vi "S2DS_Update WC (SubVI).vi"(11 "All channel parameters (in)":T1 {"Scan parameters"."Y data taking" items=["in both direction", "in up direction only", "in down direction only"]; "Scan parameters"."X data taking" items=["in both direction", "in up direction only", "in down direction only"]}) -> (2 "Change required":i32[](array[numeric]), 3 "All channel parameters (out)":T1 {"Scan parameters"."Y data taking" items=["in both direction", "in up direction only", "in down direction only"]; "Scan parameters"."X data taking" items=["in both direction", "in up direction only", "in down direction only"]})   [LabVIEW 2025]
uses:
  TYPE DEFS/S2DS_All Channel Parameters.ctl
  TYPE DEFS/S2DS_WC info.ctl
  TYPE DEFS/S2DS_Single WC info.ctl
  TYPE DEFS/S2DS_RC info.ctl
  TYPE DEFS/S2DS_Single RC info.ctl
  TYPE DEFS/S2DS_DAC info new.ctl
  TYPE DEFS/S2DS_Single DC info.ctl
  TYPE DEFS/S2DS_Array Inst Info.ctl
  TYPE DEFS/S2DS_Sweep Info.ctl
panel:
  in  "Tab Control":enum32{"Basic", "Advanced", "Formula"}(tab)
  in  "Step 2":dbl caption="Step size"
  in  "Rate up":dbl
  in  "Rate down":dbl
  in  "Min end":dbl
  in  "Max end":dbl
  in  "Data Bin size":dbl
  in  "Target 2":dbl caption="Target"
  out "Factor":dbl
  out "Current value":dbl
  in  "Factor 2":dbl
  in  "Current value 2":dbl
  out "Factor 3":dbl caption="Factor"
  out "Current value 3":dbl caption="Present level"
  in  "Update formula":bool
  in  "Undo":bool
  in  "OK 2":bool
  in  "Select channel to edit":u16(ring) items=["A ( Unit)", "A ( Unit)", "A ( Unit)", "A ( Unit)", "A ( Unit)", "A ( Unit)", "A ( Unit)", "A ( Unit)", "A ( Unit)"]
  in  "OK":bool
  # "Update Write Channel Info..."
  # "Old value"
  # "Updated"
  # "Enter new"
  # "NOTE:  If current level is not equal to target, the\nprogram will immedietely drive the instrument."
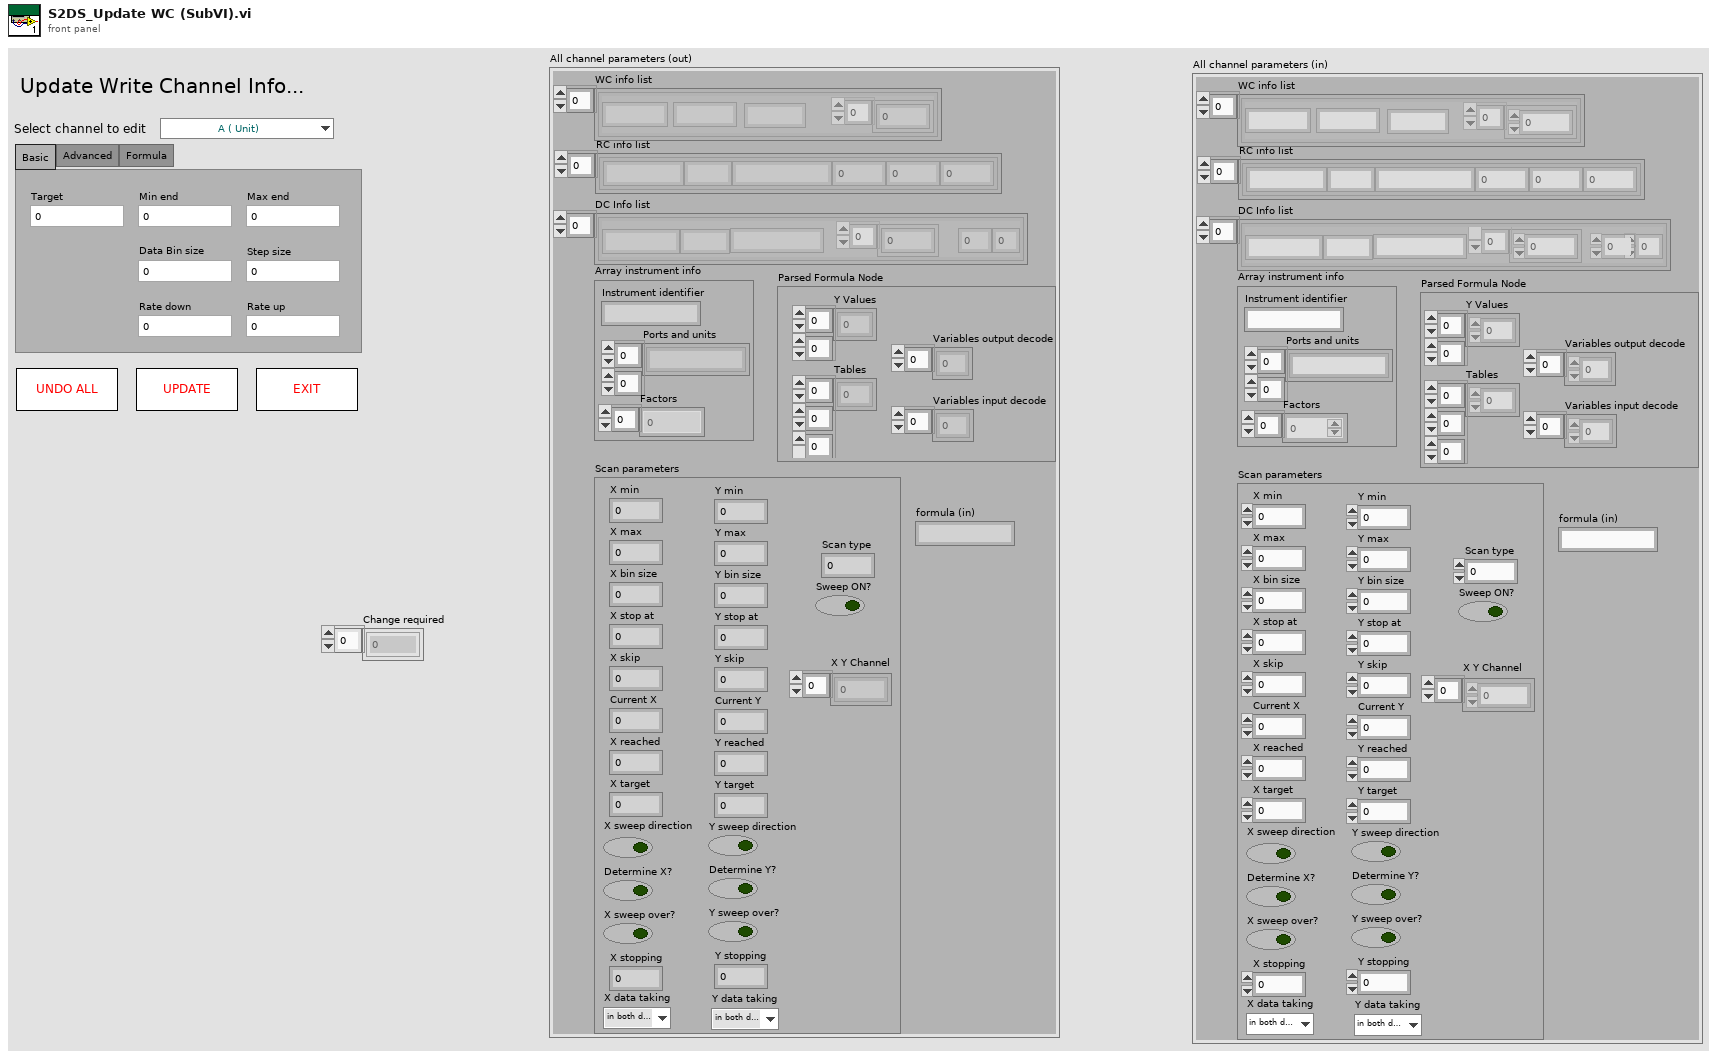
[diagram p1: front panel]
types:
  T1 = typedef "S2DS_All Channel Parameters.ctl" = cluster{"WC info list":T2, "RC info list":T4, "DC Info list":T6, "Array instrument info":T8, "Scan parameters":T9, "Parsed Formula Node":cluster{"Y Values":dbl[][], "Tables":i32[][][], "Variables input decode":i32[], "Variables output decode":i32[]}, "formula (in)":string}
  T2 = typedef "S2DS_WC info.ctl" = T3[]
  T3 = typedef "S2DS_Single WC info.ctl" = cluster{"Instrument identifier":string, "Write channel parameters":dbl[], "Name":string, "Unit":string}
  T4 = typedef "S2DS_RC info.ctl" = T5[]
  T5 = typedef "S2DS_Single RC info.ctl" = cluster{"Instrument identifier":string, "Factor":dbl, "Averaging":i32, "Wait (ms)":i32, "Unit":string, "Name":string}
  T6 = typedef "S2DS_DAC info new.ctl" = T7[]
  T7 = typedef "S2DS_Single DC info.ctl" = cluster{"Operation identifier":string, "DC parameters":dbl[], "U":i32, "V":i32, "Name":string, "Unit":string}
  T8 = typedef "S2DS_Array Inst Info.ctl" = cluster{"Instrument identifier":string, "Ports and units":string[][], "Factors":dbl[]}
  T9 = typedef "S2DS_Sweep Info.ctl" = cluster{"X min":ext, "X max":dbl, "Y min":dbl, "Y max":dbl, "X bin size":dbl, "Y bin size":dbl, "X stop at":dbl, "Y stop at":dbl, "X skip":u64, "Y skip":u64, "Current X":dbl, "Current Y":dbl, "X reached":i32, "Y reached":i32, "X target":dbl, "Y target":dbl, "Sweep ON?":bool, "X sweep direction":bool, "Y sweep direction":bool, "Determine X?":bool, "Determine Y?":bool, "X sweep over?":bool, "Y sweep over?":bool, "Scan type":i32, "X stopping":i32, "Y stopping":i32, "X Y Channel":u16[], "X data taking":u16, "Y data taking":u16}
  T10 = cluster{"Y Values":dbl[][], "Tables":i32[][][], "Variables input decode":i32[], "Variables output decode":i32[]}
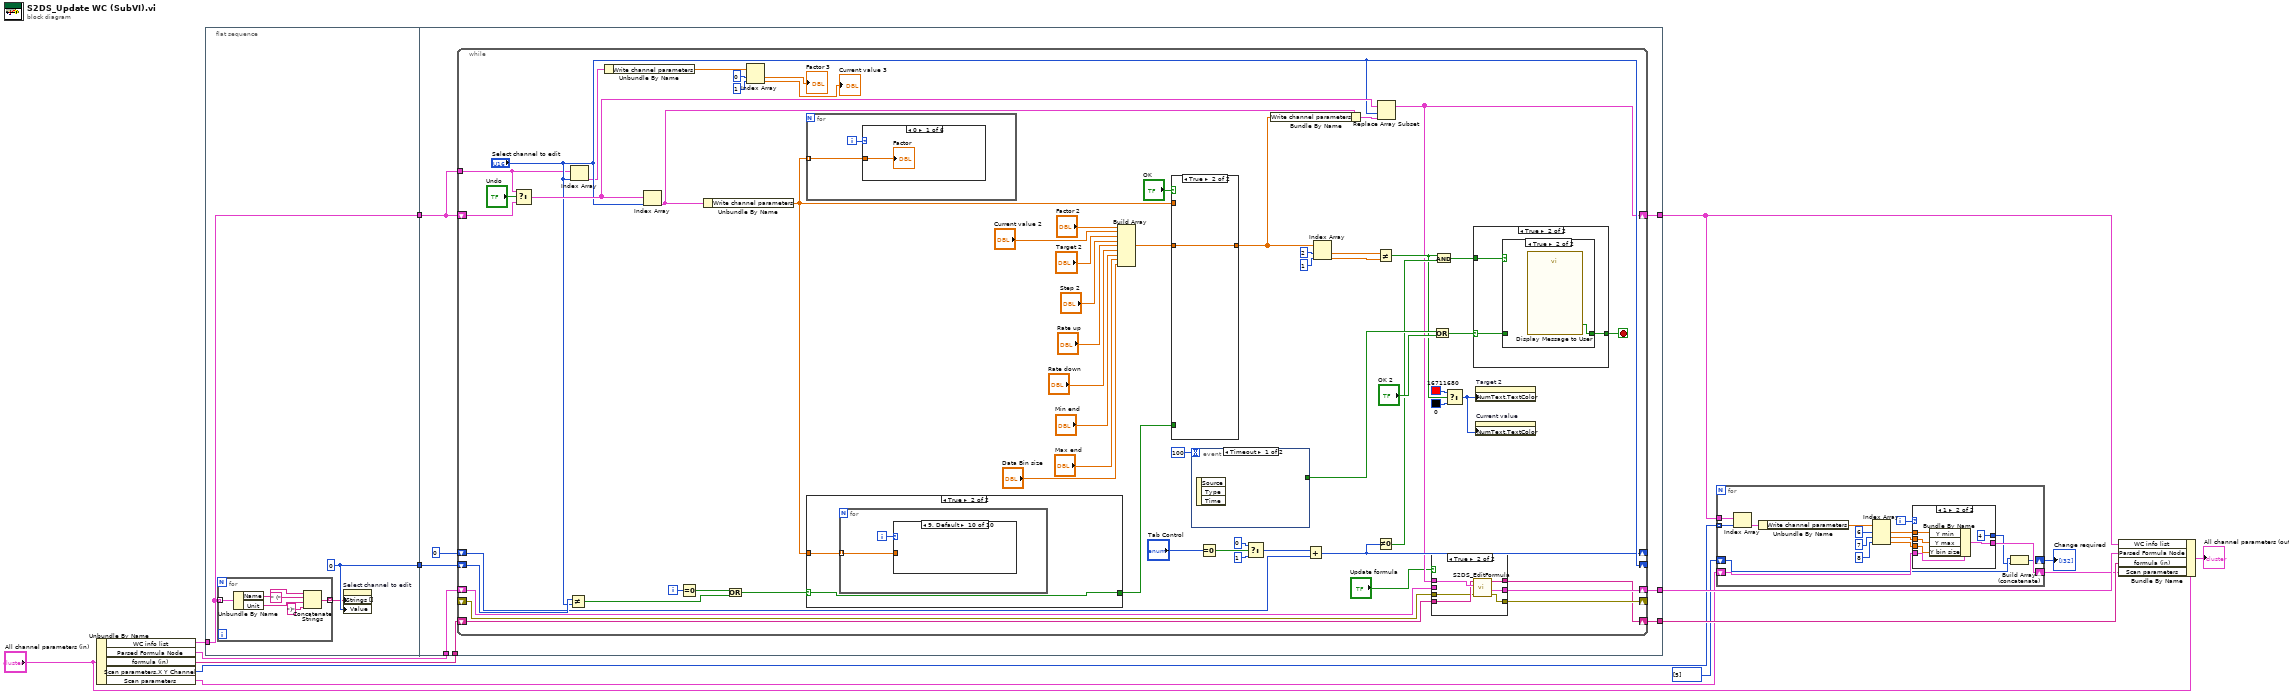
[diagram p0: block diagram]
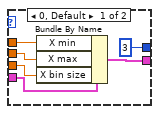
[diagram p2: hidden frame]
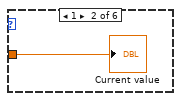
[diagram p6: hidden frame]
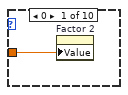
[diagram p13: hidden frame]
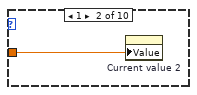
[diagram p14: hidden frame]
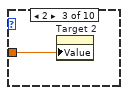
[diagram p15: hidden frame]
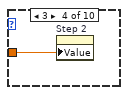
[diagram p16: hidden frame]
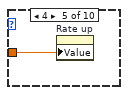
[diagram p17: hidden frame]
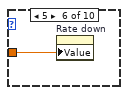
[diagram p18: hidden frame]
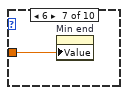
[diagram p19: hidden frame]
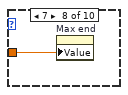
[diagram p20: hidden frame]
diagram:
  n1 = Unbundle By Name("All channel parameters (in)") -> ("WC info list"=w13:T2, "Parsed Formula Node"=w12:T10, "formula (in)"=w11:string, "Scan parameters.X Y Channel"=w6:u16[], "Scan parameters"=w4:T9)
  n2 = flat-sequence {
    tunnel: w13 -> [w17]
    tunnel: [w17] -> w15
    tunnel: [w18] -> w14
    tunnel: w15 -> [w31]
    tunnel: w14 -> [w32]
    tunnel: w12 -> [w29]
    tunnel: w11 -> [w28]
    tunnel: [w27] -> w5
    tunnel: [w26] -> w8
    tunnel: [w25] -> w7
    frame #0 {
      w18 = 0
      n3 = for {
        tunnel: w17 -> [w24] mode=indexing
        tunnel: [w19] -> w16 mode=indexing
        n4 = Unbundle By Name(w24) -> ("Name"=w23:string, "Unit"=w21:string)
        n5 = Concatenate Strings(w23, " (" ("string"), w21, ")" ("string")) -> (w19:string)
      }
      n6 = property on="Select channel to edit" class="Ring (strict)"("Strings []"=w16, "Value"=w18) -> ()  [unwired: 2 in, 2 out]
    }
    frame #1 {
      n7 = while {
        shift-right: ["Select channel to edit"] -> _
        shift-left: w32 -> [w94]
        shift-right: [w43] -> w27
        shift-left: w31 -> [w89]
        tunnel: w31 -> [w71]
        shift-right: [w47] -> _
        shift-left: 0 -> [w49]
        shift-right: [w42] -> w26
        shift-left: w29 -> [w41]
        shift-right: [w40] -> _
        shift-left: _ -> [w39]
        shift-right: [w38] -> w25
        shift-left: w28 -> [w37]
        i -> [w93]
        stop <- w54 stop-if-true
        n8 = Select(t=w71, s="Undo", f=w89) -> (s? t:f=w92:T2)
        n9 = Not Equal?(x=w94, y="Select channel to edit") -> (x != y?=w84:bool)
        n10 = Index Array(array=w71, index="Select channel to edit") -> (element=w70:T3)
        n11 = Unbundle By Name(w70) -> ("Write channel parameters"=w69:dbl[])
        n12 = Index Array(array=w92, index="Select channel to edit") -> (element=w91:T3)
        n13 = Equal To 0?(x=w93) -> (x = 0?=w83:bool)
        n14 = Unbundle By Name(w91) -> ("Write channel parameters"=w80:dbl[])
        n15 = Or(x=w83, y=w84) -> (x .or. y?=w85:bool)
        n16 = Index Array(array=w69, index #1=0 ("index"), index #2=1 ("index")) -> (element #1=→"Factor 3":dbl, element #2=→"Current value 3":dbl)
        n17 = for {
          tunnel: w80 -> [w110] mode=indexing
          i -> [w111]
          n18 = case shown="0" w111 {
            tunnel: w110 -> [w112 w113 _ _ _ _]
            frame 0 {
              "Factor" <- w112
            }
            frame 1 {
              "Current value" <- w113
            }
            frame 2 {
            }
            frame 3 {
            }
            frame 4 {
            }
            frame 5, Default {
            }
          }
        }
        n19 = case shown="True" w85 {
          selector: w85 -> [w116 w117]
          tunnel: w80 -> [_ w118]
          tunnel: [w116 w117] -> w64
          frame False {
          }
          frame True {
            n20 = for {
              tunnel: w118 -> [w119] mode=indexing
              i -> [w120]
              n21 = case shown="9, Default" w120 {
                tunnel: w119 -> [w121 w122 w123 w124 w125 w126 w127 w128 w129 _]
                frame 0 {
                  n22 = property on="Factor 2" class="DigNum (strict)"("Value"=w121) -> ()  [unwired: 2 in, 2 out]
                }
                frame 1 {
                  n23 = property on="Current value 2" class="DigNum (strict)"("Value"=w122) -> ()  [unwired: 2 in, 2 out]
                }
                frame 2 {
                  n24 = property on="Target 2" class="DigNum (strict)"("Value"=w123) -> ()  [unwired: 2 in, 2 out]
                }
                frame 3 {
                  n25 = property on="Step 2" class="DigNum (strict)"("Value"=w124) -> ()  [unwired: 2 in, 2 out]
                }
                frame 4 {
                  n26 = property on="Rate up" class="DigNum (strict)"("Value"=w125) -> ()  [unwired: 2 in, 2 out]
                }
                frame 5 {
                  n27 = property on="Rate down" class="DigNum (strict)"("Value"=w126) -> ()  [unwired: 2 in, 2 out]
                }
                frame 6 {
                  n28 = property on="Min end" class="DigNum (strict)"("Value"=w127) -> ()  [unwired: 2 in, 2 out]
                }
                frame 7 {
                  n29 = property on="Max end" class="DigNum (strict)"("Value"=w128) -> ()  [unwired: 2 in, 2 out]
                }
                frame 8 {
                  n30 = property on="Data Bin size" class="DigNum (strict)"("Value"=w129) -> ()  [unwired: 2 in, 2 out]
                }
                frame 9, Default {
                }
              }
            }
          }
        }
        n31 = Build Array("Factor 2", "Current value 2", "Target 2", "Step 2", "Rate up", "Rate down", "Min end", "Max end", "Data Bin size") -> (w73:dbl[])
        n32 = case shown="True" "OK" {
          tunnel: w73 -> [_ w115]
          tunnel: w80 -> [w114 _]
          tunnel: [w114 w115] -> w63
          tunnel: w64 -> [_ _]
          frame False {
          }
          frame True {
          }
        }
        n33 = event shown="[0] Timeout" {
          selector: _ -> [_ _]
          dyn-events: _ -> [_ _]
          timeout: 100 -> [_ _]
          tunnel: [_ w130] -> w87
          event Timeout {
            n34 = event-data() -> ()  [unwired: 1 in, 3 out]
          }
          event Panel Close? {
            w130 = TRUE ("Discard?")
            n35 = event-data() -> ()  [unwired: 1 in, 4 out]
            n36 = event-data("Discard?"=w130) -> ()  [unwired: 1 in, 1 out]
          }
        }
        n37 = Equal To 0?(x="Tab Control") -> (x = 0?=w52:bool)
        n38 = Select(t=0, s=w52, f=1) -> (s? t:f=w48:i32)
        n39 = Bundle By Name(cluster=w91, "Write channel parameters"=w63) -> (w82:T3)
        n40 = Add(x=w48, y=w49) -> (x+y=w47:i32)
        n41 = Index Array(array=w63, index #1=2 ("index"), index #2=1 ("index")) -> (element #1=w60:dbl, element #2=w59:dbl)
        n42 = Not Equal?(x=w60, y=w59) -> (x != y?=w45:bool)
        n43 = Not Equal To 0?(x=w47) -> (x != 0?=w46:bool)
        n44 = Replace Array Subset(array=w92, new element=w82, index="Select channel to edit") -> (w43:T2)
        n45 = case shown="True" "Update formula" {
          tunnel: w43 -> [_ w103]
          tunnel: [w97 w102] -> w42
          tunnel: w41 -> [w97 _]
          tunnel: [w96 w101] -> w40
          tunnel: w39 -> [w96 w98]
          tunnel: [w95 w100] -> w38
          tunnel: w37 -> [w95 w99]
          frame False {
          }
          frame True {
            n46 = call "S2DS_EditFormula.vi"("error in (no error)"=w98, "WC info out"=w103, "formula in"=w99) -> ("error out"=w101:errorcluster, "Parsed Formula Node (out)"=w102:T10, "formula (out)"=w100:string)  [unwired: 6 in]
          }
        }
        n47 = Or(x=w87, y="OK 2") -> (x .or. y?=w55:bool)
        n48 = And(x=w45, y=w46) -> (x .and. y?=w44:bool)
        n49 = Select(t=u32 16711680, s=w45, f=u32 0) -> (s? t:f=w56:u32)
        n50 = case shown="True" w55 {
          selector: w55 -> [w104 w105]
          tunnel: [w104 w107] -> w54
          tunnel: w44 -> [_ w106]
          frame False {
          }
          frame True {
            n51 = case shown="True" w106 {
              tunnel: [w108 w109] -> w107
              tunnel: w105 -> [w108 _]
              frame False {
              }
              frame True {
                n52 = call "Display Message to User"() -> ("OK"=w109:bool)  [unwired: 10 in, 1 out]
              }
            }
          }
        }
        n53 = property on="Target 2" class="DigNum (strict)"("NumText.TextColor"=w56) -> ()  [unwired: 2 in, 2 out]
        n54 = property on="Current value" class="DigNum (strict)"("NumText.TextColor"=w56) -> ()  [unwired: 2 in, 2 out]
      }
    }
  }
  n55 = for {
    tunnel: w6 -> [w145] mode=indexing
    tunnel: w5 -> [w146]
    shift-right: [w140] -> w3
    shift-left: w4 -> [w141]
    shift-right: [w131] -> w1
    shift-left: i32[] [5] -> [w133]
    i -> [w142]
    n56 = Index Array(array=w146, index=w145) -> (element=w144:T3)
    n57 = Unbundle By Name(w144) -> ("Write channel parameters"=w143:dbl[])
    n58 = Index Array(array=w143, index #1=6 ("index"), index #2=7 ("index"), index #3=8 ("index")) -> (element #1=w136:dbl, element #2=w135:dbl, element #3=w134:dbl)
    n59 = case shown="1" w142 {
      tunnel: w141 -> [w152 w158]
      tunnel: [w151 w157] -> w140
      tunnel: w136 -> [w150 w156]
      tunnel: w135 -> [w149 w155]
      tunnel: w134 -> [w148 w154]
      tunnel: [3 4] -> w132
      frame 0, Default {
        n60 = Bundle By Name(cluster=w152, "X min"=w150, "X max"=w149, "X bin size"=w148) -> (w151:T9)
      }
      frame 1 {
        n61 = Bundle By Name(cluster=w158, "Y min"=w156, "Y max"=w155, "Y bin size"=w154) -> (w157:T9)
      }
    }
    n62 = Build Array (concatenate)(w133, w132) -> (w131:i32[])
  }
  "Change required" <- w1
  n63 = Bundle By Name(cluster="All channel parameters (in)", "WC info list"=w5, "Parsed Formula Node"=w8, "formula (in)"=w7, "Scan parameters"=w3) -> (→"All channel parameters (out)":T1)
